vi "SwissSPAD Live_About.vi"() -> (11 "Version":string)   [LabVIEW 2021]
uses:
  SwissSPAD Live_Globals.vi
  Notebook/Notebook.lvlib
  Rich Text Box/Rich Text Box.lvlib
panel:
  in  "Admin Mode":bool
  in  "OK":bool
  out "SS2 Live":string="  SwissSPAD Live"
  # "© 2020-2022 The Regents of University of California\nAuthor: X. Michalet, Department of Chemistry & Biochemistry, UCLA\n\nThis software product was developed using LabVIEW™ and the National Instruments Vision Development Toolkit for LabVIEW. Funding was provided in part by grants from the US National Institute of Health (NIH) and the US Department of Energy (DOE).\n\nLabVIEW is a trademark of National Instruments.\nSwissSPAD Live is not endorsed by, or sponsored by National Instruments, NIH, DOE or UCLA. This software is provided without guaranty of any kind, whether expressed or implied."
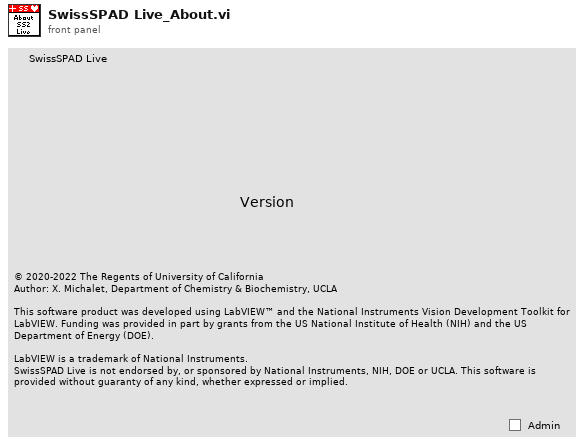
[diagram p1: front panel]
types:
  T1 = enum32{"Invalid", "Standard", "Closed", "Hidden", "Minimized", "Maximized"}
  T2 = typedef "Rich Text Box.lvlib/Text Formatting.ctl" = cluster{"Font":string, "Text Color":T3, "Text Background Color":T3, "Text Style":enum16{"Regular", "Bold", "Italic", "Underline", "Strikeout"}, "Font Size (Points)":dbl, "Text Alignment":i32}
  T3 = typedef "Rich Text Box.lvlib/Text Colors.ctl" = enum16{"Unchanged", "Black", "Blue", "Brown", "Gray", "Green", "Orange", "Pink", "Red", "White"}
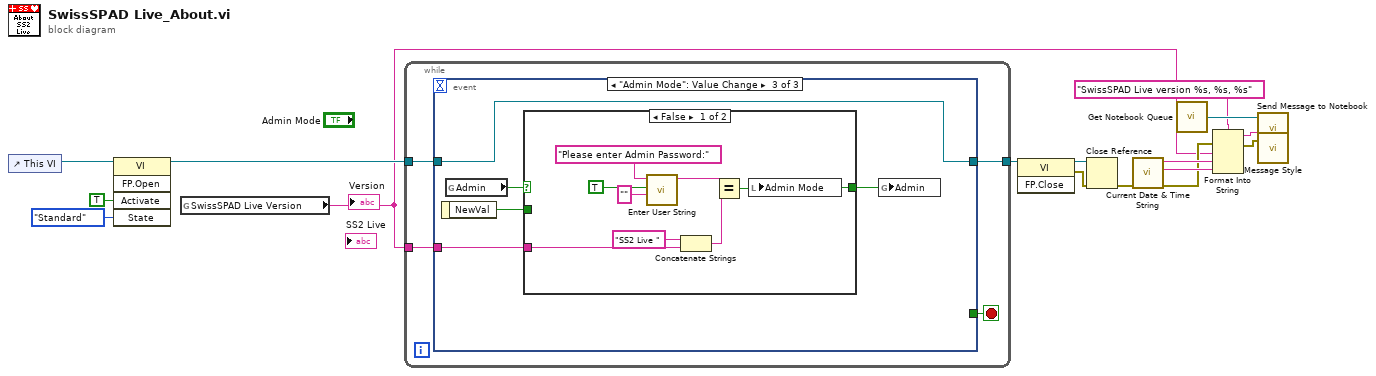
[diagram p0: block diagram]
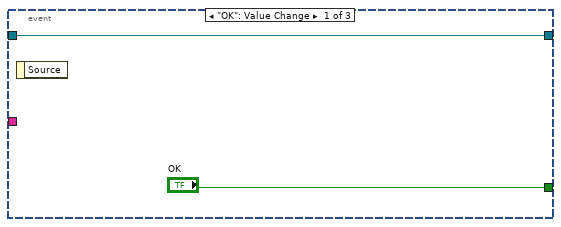
[diagram p2: hidden frame]
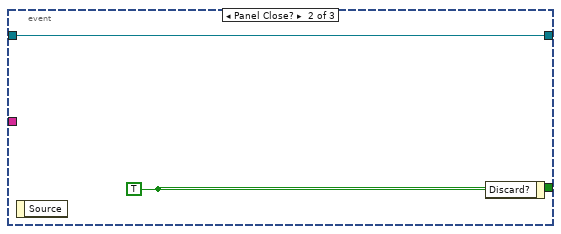
[diagram p3: hidden frame]
diagram:
  n1 = control-ref of="This VI"() -> (w15:refnum<vi>)
  n2 = invoke class="VI" method="FP.Open"(reference=w15, "Activate"=TRUE ("Activate?"), "State"=T1."Standard") -> (reference out=w14:refnum<vi>)  [unwired: 2 in, 4 out]
  n3 = global read "SwissSPAD Live_Globals.vi" "SwissSPAD Live Version"() -> (w1:string)
  "Version" <- w1
  n4 = while {
    tunnel: [w19] -> w17
    tunnel: w14 -> [w20]
    tunnel: w1 -> [w18]
    stop <- w21 stop-if-true
    n5 = event shown="[2] \"Admin Mode\": Value Change" {
      selector: _ -> [_ _ _]
      dyn-events: _ -> [_ _ _]
      timeout: _ -> [_ _ _]
      tunnel: ["OK" w25 _] -> w21
      tunnel: w20 -> [w22 w24 w29]
      tunnel: [w22 w24 w29] -> w19
      tunnel: w18 -> [_ _ w26]
      event "OK": Value Change {
        n6 = event-data() -> ()  [unwired: 1 in, 1 out]
      }
      event Panel Close? {
        w25 = TRUE ("Discard?")
        n7 = event-data() -> ()  [unwired: 1 in, 1 out]
        n8 = event-data("Discard?"=w25) -> ()  [unwired: 1 in, 1 out]
      }
      event "Admin Mode": Value Change {
        n9 = event-data() -> ("NewVal"=w28:bool)  [unwired: 1 in]
        n10 = global read "SwissSPAD Live_Globals.vi" "Admin"() -> (w30:bool)
        n11 = case shown="False" w30 {
          tunnel: w28 -> [_ w39]
          tunnel: [w35 w39] -> w27
          tunnel: w26 -> [w36 _]
          frame False {
            n12 = call "Enter User String.vi"("Caption"="" ("String Name (\"object\")"), "Clear Value (F)"=TRUE, "Message"="Please enter Admin Password:" ("Object Name in")) -> ("User entered string"=w32:string)  [unwired: 6 in, 2 out]
            n13 = Concatenate Strings("SS2 Live " ("y"), w36) -> (w37:string)
            n14 = Equal?(x=w32, y=w37) -> (x = y?=w35:bool)
            n15 = local write "Admin Mode"(w35) -> ()
          }
          frame True {
          }
        }
        n16 = global write "SwissSPAD Live_Globals.vi" "Admin"(w27) -> ()
      }
    }
  }
  n17 = invoke class="VI" method="FP.Close"(reference=w17) -> (reference out=w16:refnum<vi>, error out=w2:errorcluster)  [unwired: 2 in, 1 out]
  n18 = Close Reference(reference=w16, error in (no error)=w2) -> (error out=w3:errorcluster)
  n19 = call "Current Date & Time String.vi"("Error In"=w3) -> ("Error Out"=w9:errorcluster, "time string"=w11:string, "date string"=w10:string)  [unwired: 8 in]
  n20 = call "Get Notebook Queue.vi"() -> ("Notebook Queue"=w5:refnum<queue>)  [unwired: 9 in]
  n21 = Format Into String(format string="SwissSPAD Live version %s, %s, %s" ("initial string"), error in=w9, w1, w10, w11) -> (resulting string=w7:string, error out=w8:errorcluster)  [unwired: 1 in]
  n22 = call "Message Style.vi"() -> ("Message Formatting"=w6:T2)
  n23 = call "Send Message to Notebook.vi"("Text Formatting"=w6, "Error In"=w8, "Message"=w7, "Notebook Queue"=w5) -> ()  [unwired: 4 in, 2 out]
